vi "Convert_zrotate_line.vi"(11 "sequence line":string[](array[string])) -> (3 "command":string[](array[string]))   [LabVIEW 2017]
panel:
  in  "ダミー":string[](array[string])
  out "文字列":string
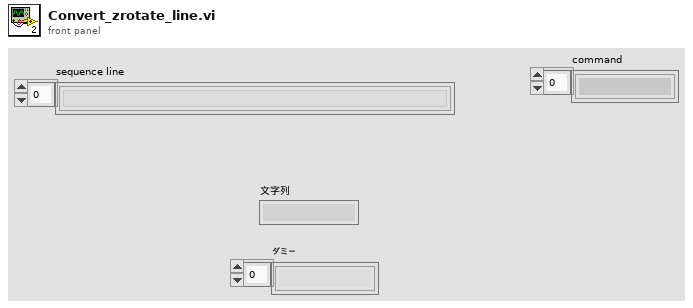
[diagram p1: front panel]
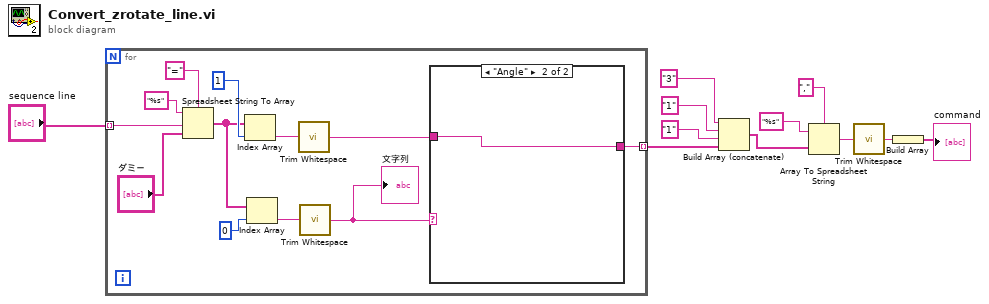
[diagram p0: block diagram]
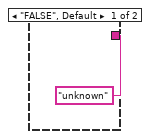
[diagram p2: hidden frame]
diagram:
  n1 = for {
    tunnel: "sequence line" -> [w23] mode=indexing
    tunnel: [w16] -> w3 mode=indexing
    n2 = Spreadsheet String To Array(delimiter (Tab)="=", format string="%s", spreadsheet string=w23, array type (2D Dbl)="ダミー") -> (array=w18:string[])
    n3 = Index Array(array=w18, index=1) -> (element=w14:string)
    n4 = Index Array(array=w18, index=0) -> (element=w15:string)
    n5 = call <vilib>:"Trim Whitespace.vi"("string"=w14) -> ("trimmed string"=w13:string)  [unwired: 1 in]
    n6 = call <vilib>:"Trim Whitespace.vi"("string"=w15) -> ("trimmed string"=w12:string)  [unwired: 1 in]
    "文字列" <- w12
    n7 = case shown="\"Angle\"" w12 {
      tunnel: w13 -> [_ w25]
      tunnel: ["unknown" w25] -> w16
      frame "FALSE", Default {
      }
      frame "Angle" {
      }
    }
  }
  n8 = Build Array (concatenate)("3", "1", "1", w3) -> (w1:string[])
  n9 = Array To Spreadsheet String(delimiter (Tab)=",", array=w1, 3:"%s") -> (spreadsheet string=w6:string)
  n10 = call <vilib>:"Trim Whitespace.vi"("string"=w6) -> ("trimmed string"=w7:string)  [unwired: 1 in]
  n11 = Build Array(w7) -> (→"command":string[])
